vi "GSF_GET.vi"(0 "Resources in":T1={"ZI Handle"={"handleValid"=FALSE, "Conn"=0, "Path Prefix"="", "Handle"=0, "Clockbase(s)"=0.0, "Connected"=FALSE}, "ZI ModHandle"={"handleValid"=FALSE, "Conn"=0, "ModHandle"=0, "moduleID"="", "Path Prefix"=""}, "VISA Keithley"="KEITHLEY"} {"ZI ModHandle"."ModHandle" format="0x%08x"; "ZI ModHandle"."Conn" format="0x%08x"; "ZI Handle"."Handle" format="0x%08x"; "ZI Handle"."Conn" format="0x%08x"}, 1 "Config files paths":T4={"ZI config file (.ini)"="Config_Ver_2\\Zurich_params.ini", "Keithley config file (.ini)"="Config_Ver_2\\Keithley_params.ini", "DAQ config file (.ini)"="Config_Ver_1\\pulse_sequence_DAQ.ini"}, 5 "AI duration (ms)":i32=100, 11 "error in":errorcluster) -> (4 "Resources out":T1 {"ZI ModHandle"."ModHandle" format="0x%08x"; "ZI ModHandle"."Conn" format="0x%08x"; "ZI Handle"."Handle" format="0x%08x"; "ZI Handle"."Conn" format="0x%08x"}, 6 "ZI DATA0 OUTPUT":cluster{"Time":dbl[], "R":dbl[]}, 8 "ZI DATA3 OUTPUT":cluster{"Time":dbl[], "R":dbl[]}, 10 "Front Data":cluster{"Time":dbl[], "Y":dbl[]}, 14 "Back Front GSF (Mean B,Mean F, SD B,SD F)":dbl[](array[numeric]), 15 "error out":errorcluster)   [LabVIEW 2021]
uses:
  Main/Ver_2/Config_File_Paths_v2.ctl
  Main/Ver_2/Resources_v2.ctl
  <instrlib>/Zurich Instruments LabOne/Public/ziTypeHandle.ctl
  <instrlib>/Zurich Instruments LabOne/Public/Modules/ziTypeModHandle.ctl
  <vilib>/Analysis/NI_AALBase.lvlib
  <instrlib>/Zurich Instruments LabOne/Zurich Instruments LabOne.lvlib
panel:
  out "Front":cluster{"Time":dbl[], "Y":dbl[]}(graph)
  out "Back Diff":dbl[](array[numeric]) format="%#_8g"
  out "ZI DATA3":cluster{"Time":dbl[], "R":dbl[]}(graph)
  out "ZI DATA0":cluster{"Time":dbl[], "R":dbl[]}(graph)
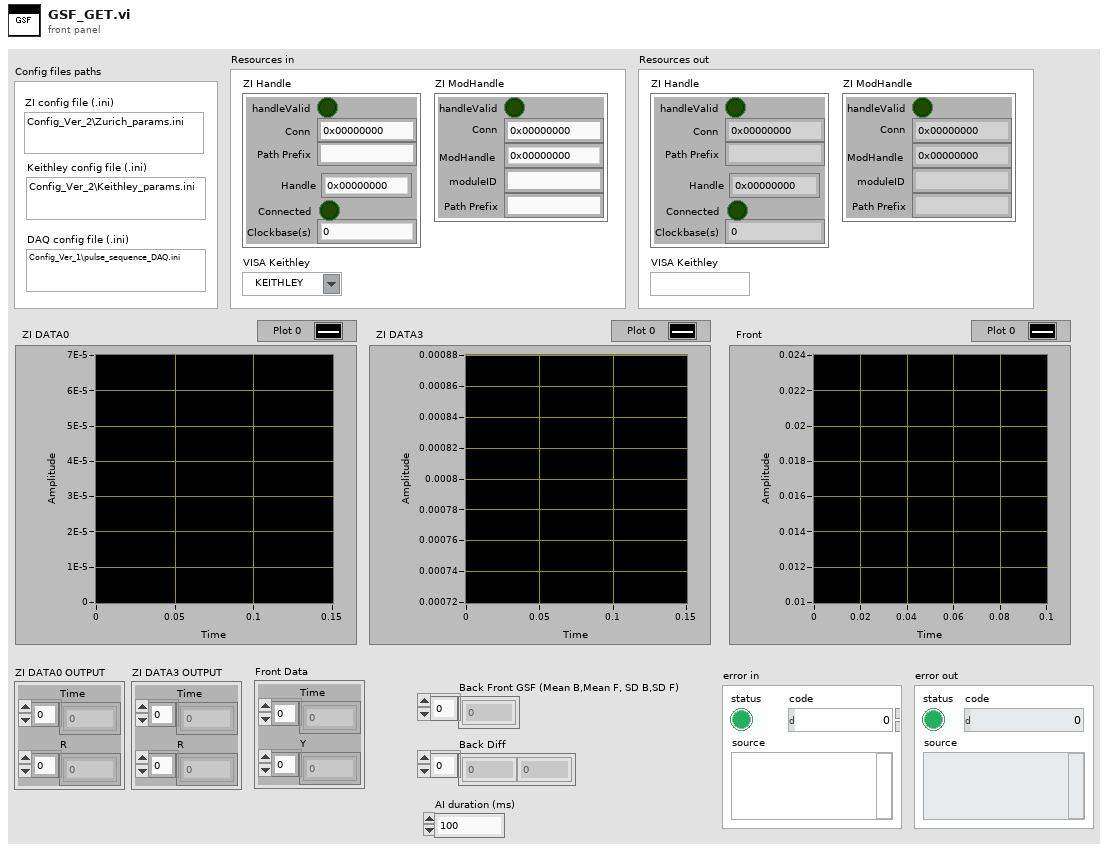
[diagram p1: front panel]
types:
  T1 = typedef "Resources_v2.ctl" = cluster{"ZI Handle":T2, "ZI ModHandle":T3, "VISA Keithley":refnum<visa-resource-name>}
  T2 = typedef "Zurich Instruments LabOne.lvlib/ziTypeHandle.ctl" = cluster{"handleValid":bool, "Conn":u64, "Path Prefix":string, "Handle":u64, "Clockbase(s)":dbl, "Connected":bool}
  T3 = typedef "Zurich Instruments LabOne.lvlib/ziTypeModHandle.ctl" = cluster{"handleValid":bool, "Conn":u64, "ModHandle":u64, "moduleID":string, "Path Prefix":string}
  T4 = typedef "Config_File_Paths_v2.ctl" = cluster{"ZI config file (.ini)":string, "Keithley config file (.ini)":string, "DAQ config file (.ini)":string}
  T5 = typedef "ZI_Data_v2.ctl" = cluster{"R":dbl[], "Theta":dbl[], "X":dbl[], "Y":dbl[], "AuxIn0":dbl[], "AuxIn1":dbl[], "Frequency":dbl[], "DIO":dbl[], "Time":dbl[]}
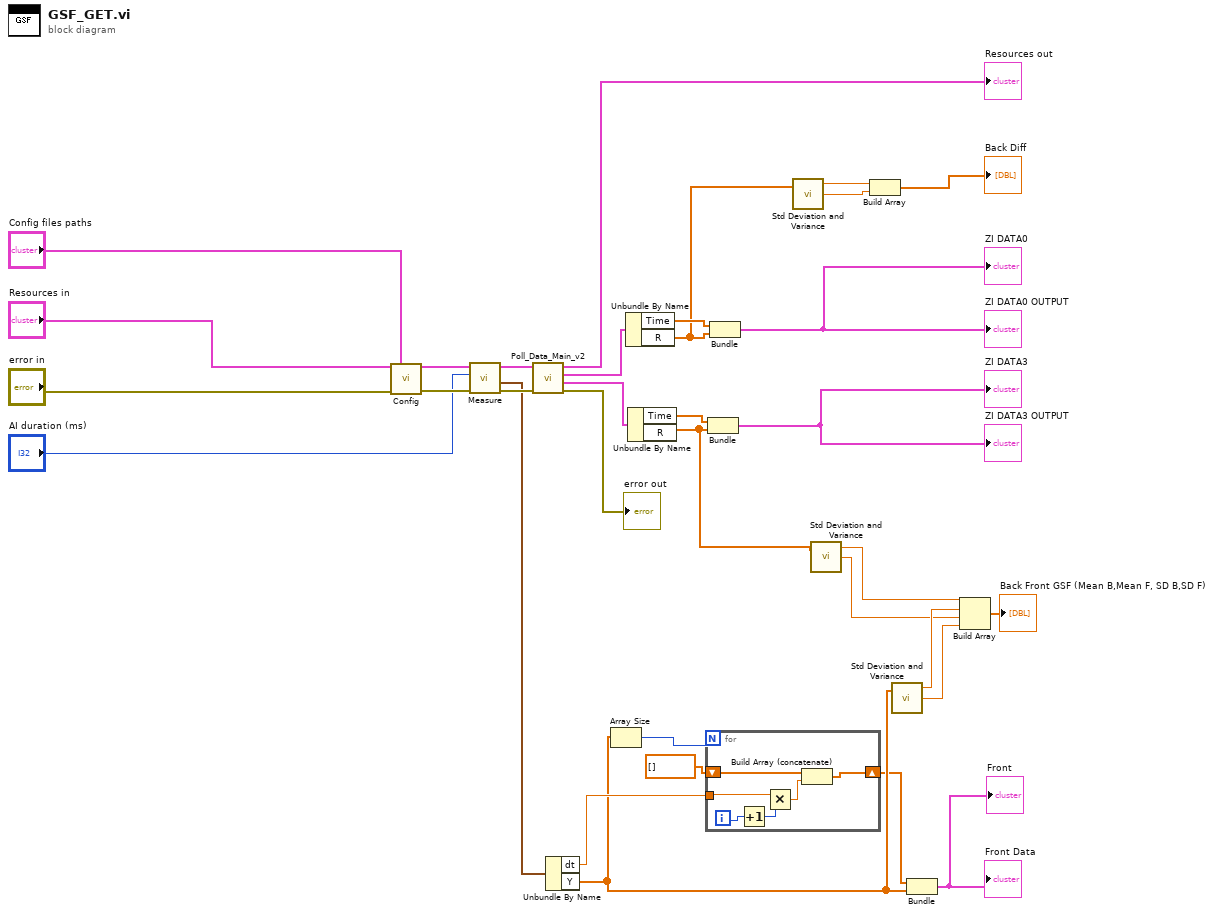
[diagram p0: block diagram]
diagram:
  n1 = call "Config.vi"("Resources in"="Resources in", "Config files paths"="Config files paths", "error in"="error in") -> ("Resources out"=w33:T1, "error out"=w32:errorcluster)  [unwired: 6 in, 5 out]
  n2 = call "Measure.vi"("error in"=w32, "AI duration (ms)"="AI duration (ms)", "Resources in"=w33) -> ("error out"=w29:errorcluster, "data"=w12:waveform(dbl), "Resources out"=w30:T1)  [unwired: 5 in, 1 out]
  n3 = call "Poll_Data_Main_v2.vi"("error in"=w29, "Resources in"=w30) -> ("error out"=→"error out":errorcluster, "ZI Data 3"=w13:T5, "ZI Data 0"=w14:T5, "Resources out"=→"Resources out":T1)  [unwired: 6 in]
  n4 = Unbundle By Name(w12) -> ("dt"=w9:dbl, "Y"=w8:dbl[])
  n5 = Array Size(array=w8) -> (size(s)=w11:i32)
  n6 = Unbundle By Name(w14) -> ("Time"=w27:dbl[], "R"=w18:dbl[])
  n7 = Unbundle By Name(w13) -> ("Time"=w25:dbl[], "R"=w15:dbl[])
  n8 = for {
    N: w11 -> [_]
    shift-right: [w34] -> w7
    shift-left: dbl[] [] ("Time") -> [w35]
    tunnel: w9 -> [w37]
    i -> [w39]
    n9 = Increment(x=w39) -> (x+1=w38:i32)
    n10 = Multiply(x=w37, y=w38) -> (x*y=w36:dbl)
    n11 = Build Array (concatenate)(w35, w36) -> (w34:dbl[])
  }
  n12 = Bundle("Time"=w25, "R"=w15) -> (→"ZI DATA3" →"ZI DATA3 OUTPUT":cluster{"Time":dbl[], "R":dbl[]})  [unwired: 1 in]
  n13 = Bundle("Time"=w27, "R"=w18) -> (→"ZI DATA0" →"ZI DATA0 OUTPUT":cluster{"Time":dbl[], "R":dbl[]})  [unwired: 1 in]
  n14 = call <vilib>:"Std Deviation and Variance.vi"("X"=w18) -> ("mean"=w17:dbl, "standard deviation"=w16:dbl)  [unwired: 1 in, 1 out]
  n15 = call <vilib>:"Std Deviation and Variance.vi"("X"=w15) -> ("mean"=w5:dbl, "standard deviation"=w3:dbl)  [unwired: 1 in, 1 out]
  n16 = Build Array(w17, w16) -> (→"Back Diff":dbl[])
  n17 = call <vilib>:"Std Deviation and Variance.vi"("X"=w8) -> ("mean"=w4:dbl, "standard deviation"=w2:dbl)  [unwired: 1 in, 1 out]
  n18 = Bundle("Time"=w7, "Y"=w8) -> (→"Front Data" →"Front":cluster{"Time":dbl[], "Y":dbl[]})  [unwired: 1 in]
  n19 = Build Array(w5, w4, w3, w2) -> (→"Back Front GSF (Mean B,Mean F, SD B,SD F)":dbl[])
